vi "letras2.vi"() -> ()   [LabVIEW 2016]
uses:
  <vilib>/Analysis/NI_AALBase.lvlib
panel:
  in  "OK Button":bool
  in  "Stop Button":bool
  out "Waveform Chart":dbl[](graph)
  out "substring":string
  out "Array":bool[](array[boolean])
  in  "String":string
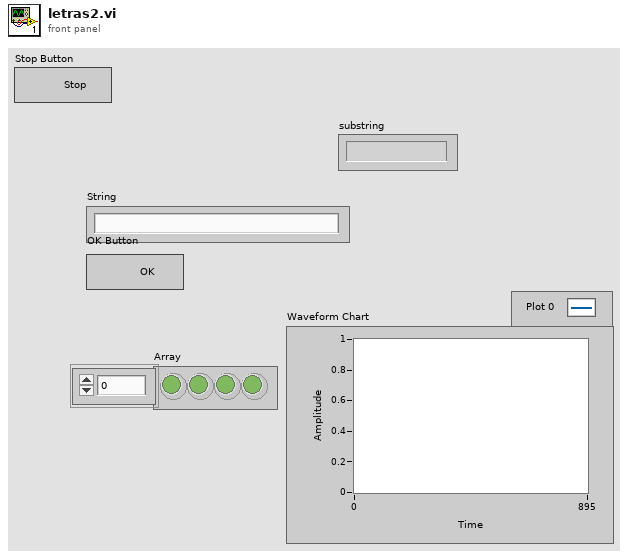
[diagram p1: front panel]
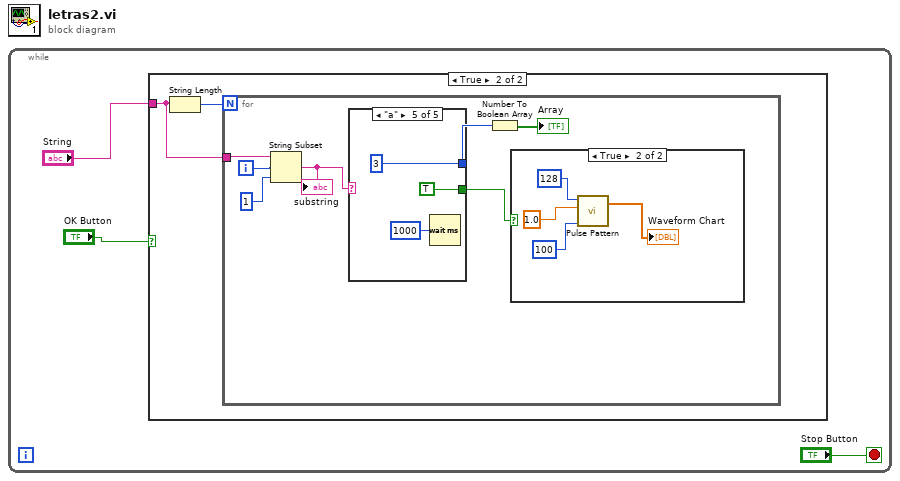
[diagram p0: block diagram]
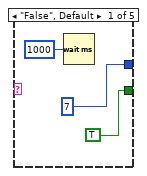
[diagram p4: hidden frame]
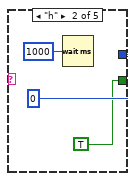
[diagram p5: hidden frame]
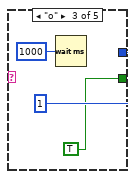
[diagram p6: hidden frame]
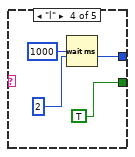
[diagram p7: hidden frame]
diagram:
  n1 = while {
    stop <- "Stop Button" stop-if-true
    n2 = case shown="True" "OK Button" {
      tunnel: "String" -> [_ w5]
      frame False {
      }
      frame True {
        n3 = String Length(string=w5) -> (length=w4:i32)
        n4 = for {
          N: w4 -> [_]
          tunnel: w5 -> [w12]
          i -> [w10]
          n5 = String Subset(string=w12, offset (0)=w10, length (rest)=1 ("length (rest)")) -> (substring=w9:string)
          "substring" <- w9
          n6 = case shown="\"a\"" w9 {
            tunnel: [7 0 1 2 3] -> w8
            tunnel: [TRUE TRUE TRUE TRUE TRUE] -> w6
            frame "False", Default {
              n7 = Wait (ms)(milliseconds to wait=u32 1000) -> ()  [unwired: 1 out]
            }
            frame "h" {
              n8 = Wait (ms)(milliseconds to wait=u32 1000) -> ()  [unwired: 1 out]
            }
            frame "o" {
              n9 = Wait (ms)(milliseconds to wait=u32 1000) -> ()  [unwired: 1 out]
            }
            frame "l" {
              n10 = Wait (ms)(milliseconds to wait=u32 1000) -> ()  [unwired: 1 out]
            }
            frame "a" {
              n11 = Wait (ms)(milliseconds to wait=u32 1000) -> ()  [unwired: 1 out]
            }
          }
          n12 = Number To Boolean Array(number=w8) -> (Boolean array=→"Array":bool[])
          n13 = case shown="True" w6 {
            frame False {
            }
            frame True {
              n14 = call <vilib>:"Pulse Pattern.vi"("width"=100, "amplitude"=1.0, "samples"=128) -> ("Pulse Pattern"=→"Waveform Chart":dbl[])  [unwired: 1 in, 1 out]
            }
          }
        }
      }
    }
  }
